vi "extracted create string buffer.vi"(8 "error in":errorcluster, 10 "Buffer Size (1024)":i32=1024) -> (0 "error out":errorcluster, 2 "dub Buffer Size":i32=1024, 3 "String Buffer":string)   [LabVIEW 2026, in "Nominal Core Streaming Engine.lvlib"]
uses:
  Nominal Core Streaming Engine.lvlib
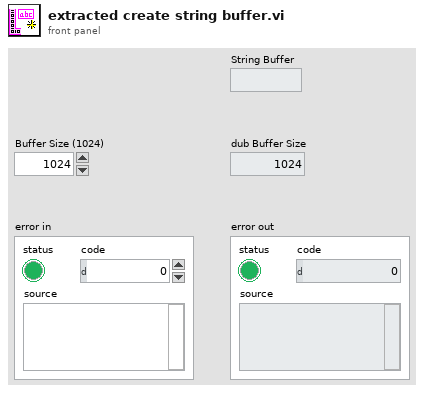
[diagram p1: front panel]
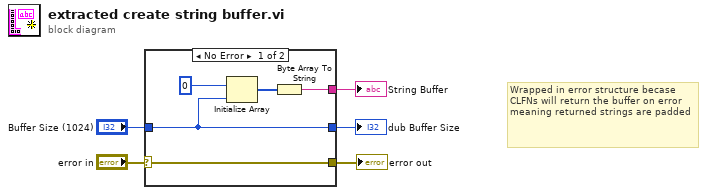
[diagram p0: block diagram]
diagram:
  # "Wrapped in error structure becase CLFNs will return the buffer on error meaning returned strings are padded"
  n1 = case shown="No Error" "error in" {
    selector: "error in" -> [w6 w12]
    tunnel: [w8 _] -> w5
    tunnel: "Buffer Size (1024)" -> [w7 w11]
    tunnel: [w6 w12] -> w2
    tunnel: [w7 w11] -> w1
    frame No Error {
      n2 = Initialize Array(u8 0, w7) -> (w9:u8[])
      n3 = Byte Array To String(unsigned byte array=w9) -> (string=w8:string)
    }
    frame Error {
    }
  }
  "String Buffer" <- w5
  "dub Buffer Size" <- w1
  "error out" <- w2
